vi "jan27_2016.vi"(8 "Image 2":T3(plugin-control)=refnum, 9 "Sequence Storer 2":T1[][](array[typedef]) {"Amplitude Correction" step=0.1; "Line Trapping"."Phase Gradient" step=0.05; "Line Trapping"."Vector"."x" step=1e-06 format="%#_6p"; "Line Trapping"."Vector"."y" step=1e-06 format="%#_6p"; "Line Trapping"."Vector"."z" step=1e-06 format="%#_6p"; "NA Position"."r" step=1e-06; "NA Position"."y" step=1e-06; "NA Position"."x" step=1e-06; "Position"."z" step=1e-06; "Position"."y" step=1e-06; "Position"."x" step=1e-06; "Phase" step=0.7753; "Intensity" step=0.1}, 10 "Total Frames":dbl, 11 "Sequence Storer":T1[][](array[typedef]) {"Amplitude Correction" step=0.1; "Line Trapping"."Phase Gradient" step=0.05; "Line Trapping"."Vector"."x" step=1e-06 format="%#_6p"; "Line Trapping"."Vector"."y" step=1e-06 format="%#_6p"; "Line Trapping"."Vector"."z" step=1e-06 format="%#_6p"; "NA Position"."r" step=1e-06; "NA Position"."y" step=1e-06; "NA Position"."x" step=1e-06; "Position"."z" step=1e-06; "Position"."y" step=1e-06; "Position"."x" step=1e-06; "Phase" step=0.7753; "Intensity" step=0.1}) -> ()   [LabVIEW 2015]
uses:
  subvis/spot.ctl
  subvis/line_trapping.ctl
panel:
  out "Position":cluster{"x":dbl, "y":dbl, "z":dbl}
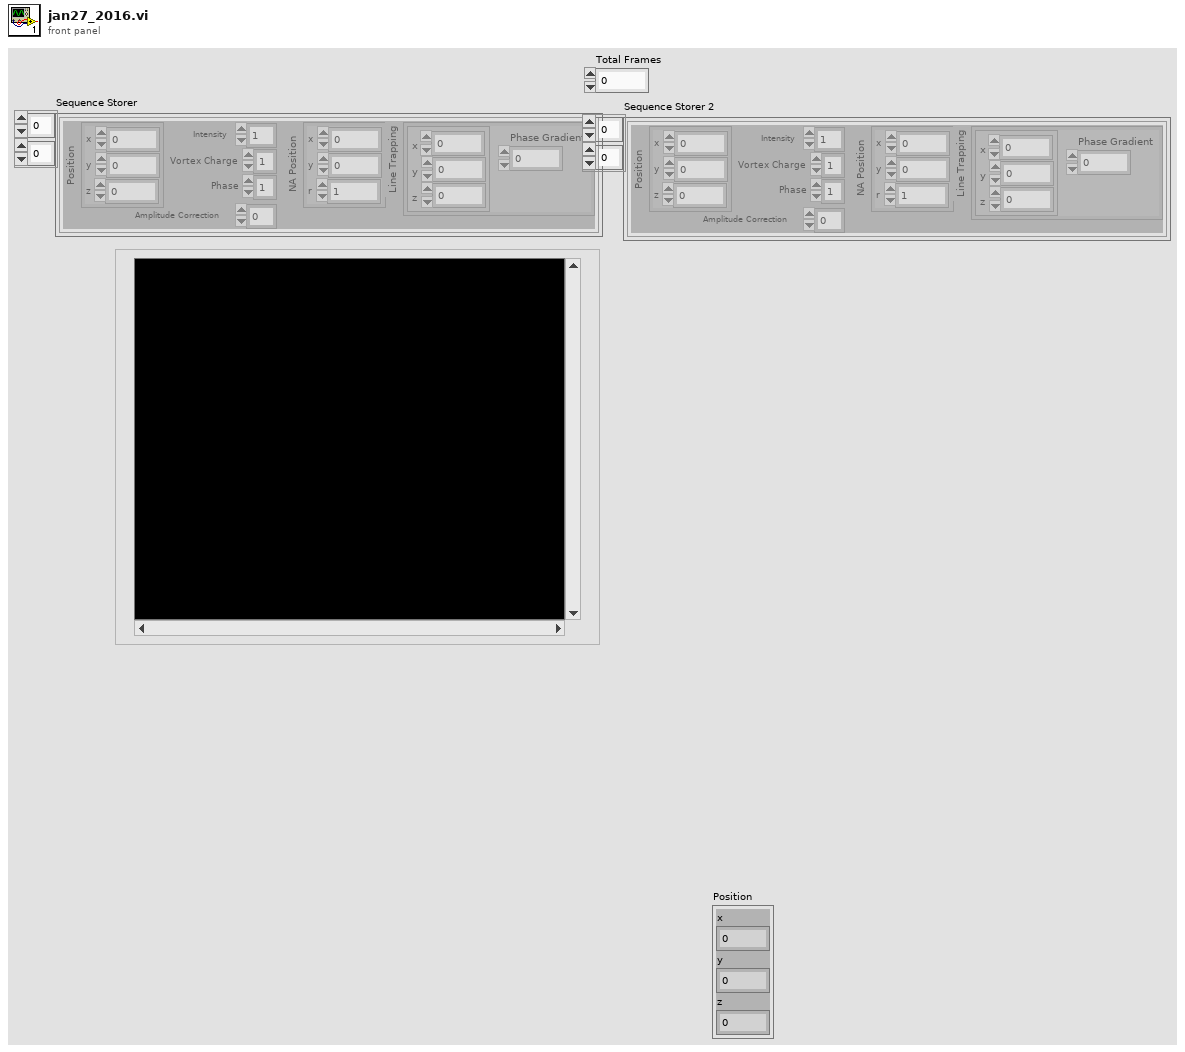
[diagram p1: front panel]
types:
  T1 = typedef "spot.ctl" = cluster{"Position":cluster{"x":dbl, "y":dbl, "z":dbl}, "Intensity":dbl, "Vortex Charge":i8, "Phase":dbl, "NA Position":cluster{"x":dbl, "y":dbl, "r":dbl}, "Line Trapping":T2, "Amplitude Correction":dbl}
  T2 = typedef "line_trapping.ctl" = cluster{"Vector":cluster{"x":dbl, "y":dbl, "z":dbl}, "Phase Gradient":dbl}
  T3 = typedef "IMAQ Image.ctl" = refnum<image>
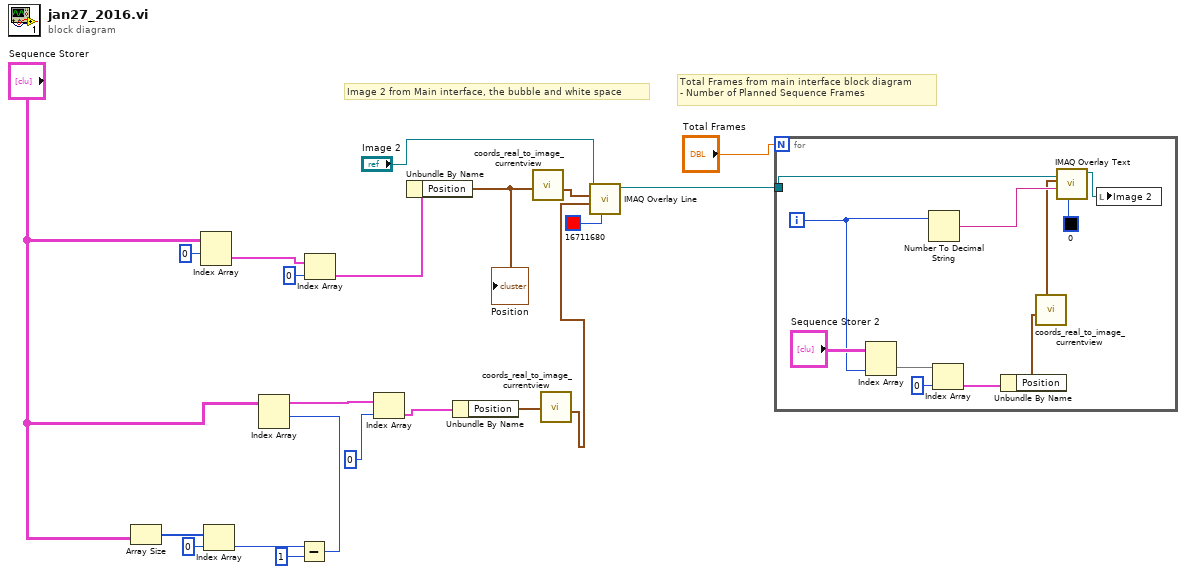
[diagram p0: block diagram]
diagram:
  # "Total Frames from main interface block diagram\n- Number of Planned Sequence Frames"
  # "Image 2 from Main interface, the bubble and white space"
  n1 = Array Size(array="Sequence Storer") -> (size(s)=w18:i32[])
  n2 = Index Array(array="Sequence Storer", index (row)=0) -> (element=w16:T1[])  [unwired: 1 in]
  n3 = Index Array(array=w18, index=0) -> (element=w10:i32)
  n4 = Subtract(x=w10, y=1) -> (x-y=w6:i32)
  n5 = Index Array(array="Sequence Storer", index (row)=w6) -> (element=w17:T1[])  [unwired: 1 in]
  n6 = Index Array(array=w16, index=0) -> (element=w12:T1)
  n7 = Index Array(array=w17, index=0) -> (element=w5:T1)
  n8 = Unbundle By Name(w12) -> ("Position"=w7:cluster{"x":dbl, "y":dbl, "z":dbl})
  "Position" <- w7
  n9 = Unbundle By Name(w5) -> ("Position"=w4:cluster{"x":dbl, "y":dbl, "z":dbl})
  n10 = call "coords_real_to_image_currentview.vi"("Position (real coords)"=w7) -> ("Position (pixels, relative to the top left of the image)"=w19:cluster{dbl, dbl})  [unwired: 7 in, 1 out]
  n11 = call "coords_real_to_image_currentview.vi"("Position (real coords)"=w4) -> ("Position (pixels, relative to the top left of the image)"=w1:cluster{dbl, dbl})  [unwired: 7 in, 1 out]
  n12 = call "IMAQ Overlay Line"("Color"=u32 16711680, "End Point"=w1, "Start Point"=w19, "Image"="Image 2") -> ("Image Out"=w20:T3)  [unwired: 6 in, 1 out]
  n13 = for {
    N: "Total Frames" -> [_]
    tunnel: w20 -> [w23]
    i -> [w28]
    n14 = Index Array(array="Sequence Storer 2", index (row)=w28) -> (element=w32:T1[])  [unwired: 1 in]
    n15 = Number To Decimal String(number=w28) -> (decimal integer string=w27:string)  [unwired: 1 in]
    n16 = Index Array(array=w32, index=0) -> (element=w29:T1)
    n17 = Unbundle By Name(w29) -> ("Position"=w25:cluster{"x":dbl, "y":dbl, "z":dbl})
    n18 = call "coords_real_to_image_currentview.vi"("Position (real coords)"=w25) -> ("Position (pixels, relative to the top left of the image)"=w24:cluster{dbl, dbl})  [unwired: 7 in, 1 out]
    n19 = call "IMAQ Overlay Text"("Text Color (black)"=u32 0, "String"=w27, "Origin"=w24, "Image"=w23) -> ("Image Out"=w22:T3)  [unwired: 6 in, 1 out]
    n20 = local write "Image 2"(w22) -> ()
  }
